vi "Delay with Cancel no error.vi"(6 "Insert Error":bool, 8 "error in (no error)":errorcluster, 11 "Delay(s)":dbl) -> (0 "error out":errorcluster, 2 "Cancelled":bool)   [LabVIEW 2018]
uses:
  Main/Main Globals.vi
  Utilities.lvlib
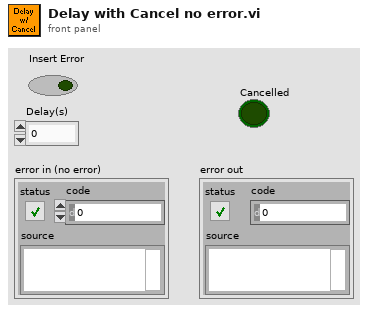
[diagram p1: front panel]
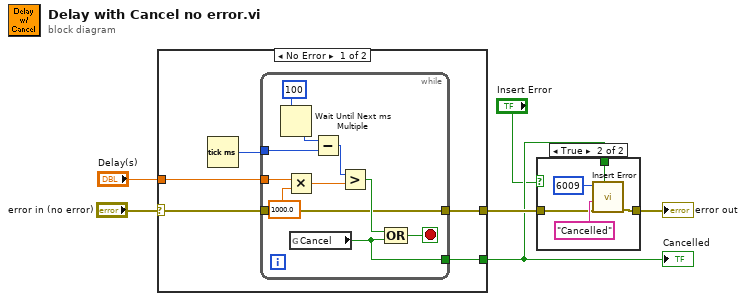
[diagram p0: block diagram]
diagram:
  n1 = case shown="No Error" "error in (no error)" {
    selector: "error in (no error)" -> [w8 w23]
    tunnel: "Delay(s)" -> [w11 _]
    tunnel: [w10 w23] -> w4
    tunnel: [w9 _] -> w2
    frame No Error {
      n2 = Tick Count (ms)() -> (millisecond timer value=w7:u32)
      n3 = while {
        tunnel: w8 -> [w17]
        tunnel: [w17] -> w10
        tunnel: w11 -> [w16]
        tunnel: [w15] -> w9
        tunnel: w7 -> [w12]
        stop <- w18 stop-if-true
        n4 = Wait Until Next ms Multiple(millisecond multiple=u32 100) -> (millisecond timer value=w13:u32)
        n5 = Multiply(x=w16, y=1000.0) -> (x*y=w20:dbl)
        n6 = global read "Main Globals.vi" "Cancel"() -> (w15:bool)
        n7 = Subtract(x=w13, y=w12) -> (x-y=w14:u32)
        n8 = Greater?(x=w14, y=w20) -> (0:w19:bool)
        n9 = Compound Arithmetic op=OR(w19, w15) -> (w18:bool)
      }
    }
    frame Error {
    }
  }
  "Cancelled" <- w2
  n10 = case shown="True" "Insert Error" {
    tunnel: w4 -> [w24 w27]
    tunnel: [w24 w26] -> w3
    tunnel: w2 -> [_ w25]
    frame False {
    }
    frame True {
      n11 = call "Insert Error.vi"("[error code] (0)"=6009, "error description"="Cancelled", "error in (no error)"=w27, "error?"=w25) -> ("error out"=w26:errorcluster)  [unwired: 6 in]
    }
  }
  "error out" <- w3
